vi "Autonomous Independent.vi"() -> ()   [LabVIEW 2013]
doc: "This VI is called when autonomous begins, and will automatically be terminated when autonomous ends. You can carry out timed or sensor driven robot movement independently without needing to return to the caller."
uses:
  TankDriveEnum.ctl
  Robot Global Data.vi
panel:
  out "Hot?":bool
  in  "Drive?":bool
  in  "DesiredMotorInput":dbl=0.4
  in  "% Cutoff":dbl=0.5
  in  "Num samples":i32=5
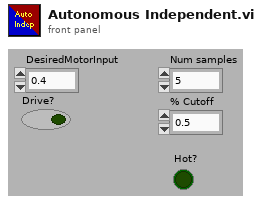
[diagram p1: front panel]
types:
  T1 = typedef "TankDriveEnum.ctl" = enum16{"Init", "LinearDrive", "SetValue", "Disable"}
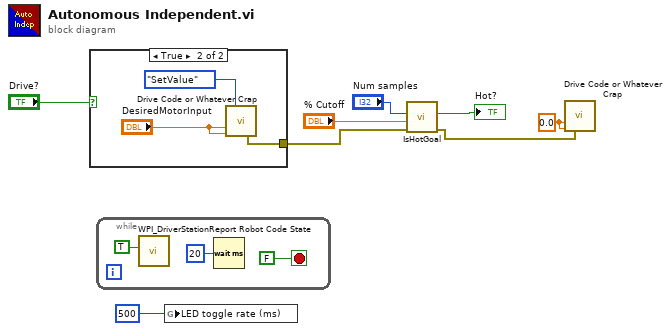
[diagram p0: block diagram]
diagram:
  w3 = 0.0 ("RightDesired")
  n1 = case shown="True" "Drive?" {
    tunnel: [_ w11] -> w5
    frame False {
    }
    frame True {
      n2 = call "Drive Code or Whatever Crap.vi"("TankDriveEnum"=TankDriveEnum."SetValue", "RightDesired"="DesiredMotorInput", "LeftDesired"="DesiredMotorInput") -> ("error out"=w11:errorcluster)  [unwired: 10 in, 2 out]
    }
  }
  n3 = while {
    stop <- FALSE stop-if-true
    n4 = call <vilib>:"WPI_DriverStationReport Robot Code State.vi"("Autonomous"=TRUE) -> ()  [unwired: 10 in, 1 out]
    n5 = Wait (ms)(milliseconds to wait=u32 20) -> ()  [unwired: 1 out]
  }
  n6 = global write "Robot Global Data.vi" "LED toggle rate (ms)"(u32 500 ("LED ms toggle rate")) -> ()
  n7 = call "IsHotGoal.vi"("error in"=w5, "% Cutoff"="% Cutoff", "Num samples"="Num samples") -> ("error out"=w2:errorcluster, "Hot/Not"=→"Hot?":bool)  [unwired: 7 in]
  n8 = call "Drive Code or Whatever Crap.vi"("RightDesired"=w3, "LeftDesired"=w3, "error in (no error)"=w2) -> ()  [unwired: 10 in, 3 out]
